vi "DSF.Engine.Pool.ID.Destroy.vi"(8 "error in (no error)":errorcluster, 11 "ID Pool in":refnum<class "DSF.Engine.Pool.ID.lvclass">) -> (0 "error out":errorcluster, 3 "ID Pool out":refnum<class "DSF.Engine.Pool.ID.lvclass">)   [LabVIEW 2017, in "DSF.Engine.lvlib" / "DSF.Engine.Pool.ID.lvclass"]
uses:
  DSF.Engine.Pool.ID.lvclass
  C:/Git/DSF/Source/Engine/Classes/Thread Pool/DSF.Engine.Pool.lvclass
  DSF.Engine.Pool.lvclass
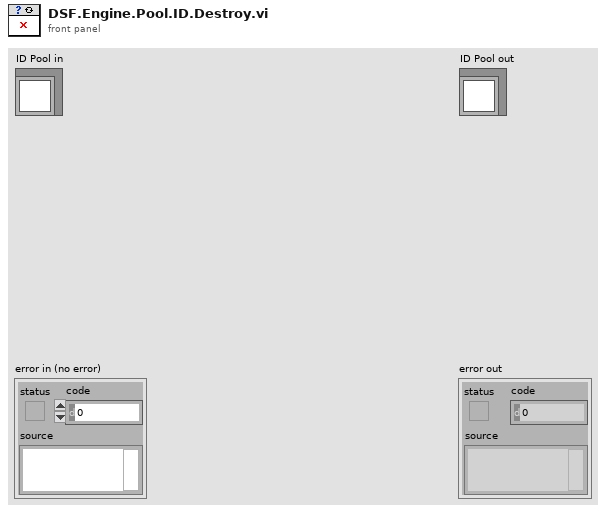
[diagram p1: front panel]
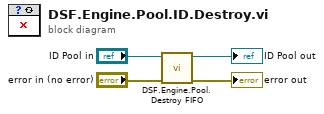
[diagram p0: block diagram]
diagram:
  n1 = call "DSF.Engine.Pool.Destroy FIFO.vi"("error in (no error)"="error in (no error)", "Pool in"="ID Pool in") -> ("error out"=→"error out":errorcluster, "Pool out"=→"ID Pool out":refnum<class "DSF.Engine.Pool.ID.lvclass">)  [unwired: 8 in]
